vi "verificador de numeros.vi"() -> ()   [LabVIEW 2020]
panel:
  out "# Interactions":dbl
  out "Current number":dbl
  in  "Number to match":dbl
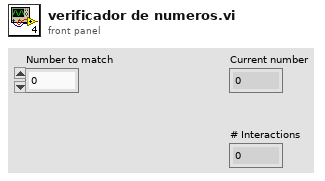
[diagram p1: front panel]
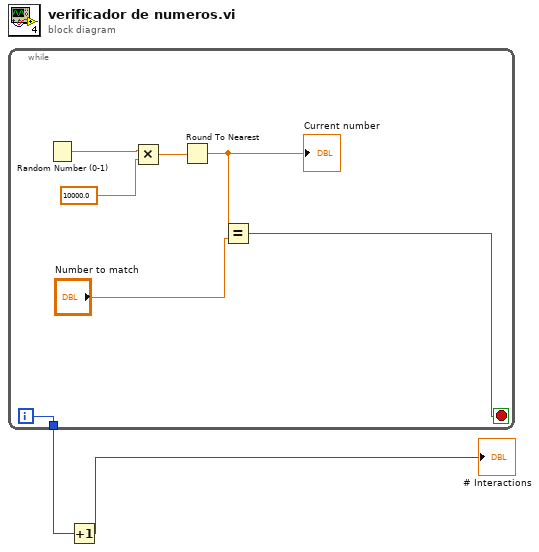
[diagram p0: block diagram]
diagram:
  n1 = while {
    tunnel: [w3] -> w1
    i -> [w3]
    stop <- w4 stop-if-true
    n2 = Random Number (0-1)() -> (number: 0 to 1=w8:dbl)
    n3 = Multiply(x=w8, y=10000.0 ("number (0 to 1)")) -> (x*y=w7:dbl)
    n4 = Round To Nearest(number=w7) -> (nearest integer value=w5:dbl)
    "Current number" <- w5
    n5 = Equal?(x=w5, y="Number to match") -> (x = y?=w4:bool)
  }
  n6 = Increment(x=w1) -> (x+1=→"# Interactions":i32)
